vi "Auton_Sr_Shoot_Move_6B.vi"   [LabVIEW 2019]
uses:
  Robot Global Data.vi
types:
  T1 = typedef "CTRE_PigeonIMU_DeviceRef.ctl" = cluster{"DeviceStatus":errorcluster, "Device Number":u8, "Type":T2, "Device ID":u32, "Handle":u64, "UsageFrame":u32, "Library Path":path}
  T2 = typedef "CTRE_PigeonIMU_ConnectionType.ctl" = u32
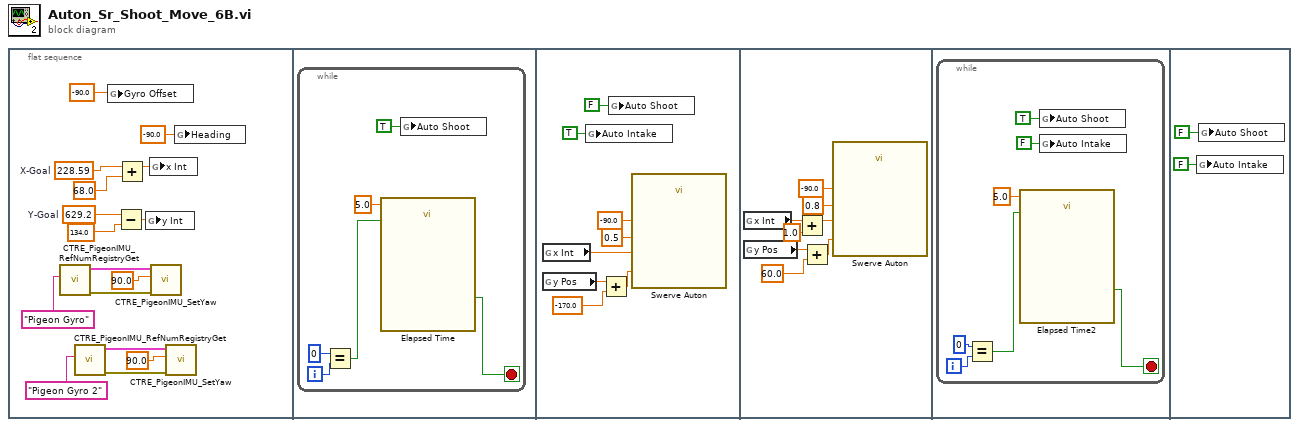
[diagram p0: block diagram]
diagram:
  n1 = flat-sequence {
    frame #0 {
      w16 = 228.59  # X-Goal
      w14 = 629.2  # Y-Goal
      n2 = call <vilib>:"CTRE_PigeonIMU_RefNumRegistryGet.vi"("refnum name"="Pigeon Gyro") -> ("error out"=w10:errorcluster, "PigeonIMUDevRef"=w9:T1)  [unwired: 9 in]
      n3 = call <vilib>:"CTRE_PigeonIMU_RefNumRegistryGet.vi"("refnum name"="Pigeon Gyro 2") -> ("error out"=w6:errorcluster, "PigeonIMUDevRef"=w5:T1)  [unwired: 9 in]
      n4 = global write "Robot Global Data.vi" "Gyro Offset"(-90.0 ("Auto Y")) -> ()
      n5 = Subtract(x=w14, y=134.0) -> (x-y=w15:dbl)
      n6 = Add(x=w16, y=68.0) -> (x+y=w12:dbl)
      n7 = global write "Robot Global Data.vi" "y Int"(w15) -> ()
      n8 = global write "Robot Global Data.vi" "x Int"(w12) -> ()
      n9 = call <vilib>:"CTRE_PigeonIMU_SetYaw.vi"("error in (no error)"=w10, "Value"=90.0, "PigeonIMUDevRef"=w9) -> ()  [unwired: 7 in, 2 out]
      n10 = call <vilib>:"CTRE_PigeonIMU_SetYaw.vi"("error in (no error)"=w6, "Value"=90.0, "PigeonIMUDevRef"=w5) -> ()  [unwired: 7 in, 2 out]
      n11 = global write "Robot Global Data.vi" "Heading"(-90.0 ("Heading")) -> ()
    }
    frame #1 {
      n12 = while {
        i -> [w18]
        stop <- w21 stop-if-true
        n13 = Equal?(x=0, y=w18) -> (x = y?=w17:bool)
        n14 = call "Elapsed Time"("Time Target (s)"=5.0, "Reset"=w17) -> ("Time has Elapsed"=w21:bool)  [unwired: 10 in, 7 out]
        n15 = global write "Robot Global Data.vi" "Auto Shoot"(TRUE ("Auto Shoot")) -> ()
      }
    }
    frame #2 {
      n16 = global read "Robot Global Data.vi" "x Int"() -> (w23:dbl)
      n17 = global read "Robot Global Data.vi" "y Pos"() -> (w27:dbl)
      n18 = global write "Robot Global Data.vi" "Auto Intake"(TRUE ("Auto Shoot")) -> ()
      n19 = Add(x=w27, y=-170.0 ("y Distance")) -> (x+y=w26:dbl)
      n20 = global write "Robot Global Data.vi" "Auto Shoot"(FALSE ("Auto Shoot")) -> ()
      n21 = call "Swerve Auton.vi"("Heading"=-90.0, "y Distance"=w26, "x Distance"=w23, "Power"=0.5) -> ()  [unwired: 8 in]
    }
    frame #3 {
      n22 = global read "Robot Global Data.vi" "x Int"() -> (w33:dbl)
      n23 = global read "Robot Global Data.vi" "y Pos"() -> (w36:dbl)
      n24 = Add(x=w33, y=1.0) -> (x+y=w32:dbl)
      n25 = Add(x=w36, y=60.0 ("y Distance")) -> (x+y=w35:dbl)
      n26 = call "Swerve Auton.vi"("Heading"=-90.0, "y Distance"=w35, "x Distance"=w32, "Power"=0.8) -> ()  [unwired: 8 in]
    }
    frame #4 {
      n27 = while {
        i -> [w40]
        stop <- w44 stop-if-true
        n28 = Equal?(x=0, y=w40) -> (x = y?=w39:bool)
        n29 = call "Elapsed Time2"("Time Target (s)"=5.0, "Reset"=w39) -> ("Time has Elapsed"=w44:bool)  [unwired: 10 in, 7 out]
        n30 = global write "Robot Global Data.vi" "Auto Shoot"(TRUE ("Auto Shoot")) -> ()
        n31 = global write "Robot Global Data.vi" "Auto Intake"(FALSE ("Auto Shoot")) -> ()
      }
    }
    frame #5 {
      n32 = global write "Robot Global Data.vi" "Auto Intake"(FALSE ("Auto Shoot")) -> ()
      n33 = global write "Robot Global Data.vi" "Auto Shoot"(FALSE ("Auto Shoot")) -> ()
    }
  }
